vi "SI SetVoltage.vi"(8 "error in (no error)":errorcluster, 10 "Voltage":dbl, 11 "VISA Refnum in":refnum<visa-resource-name>) -> (0 "error out":errorcluster, 3 "String":string)   [LabVIEW 2017]
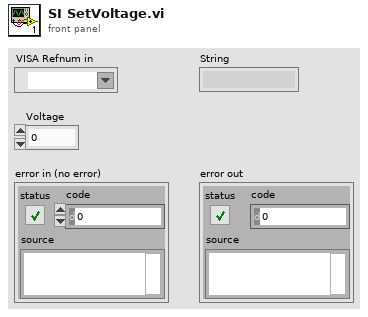
[diagram p1: front panel]
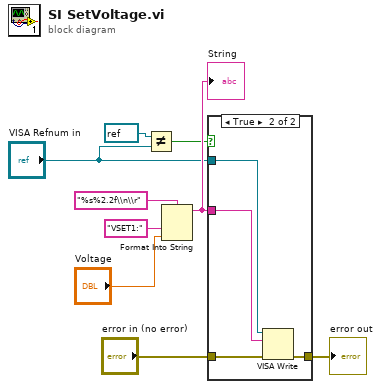
[diagram p0: block diagram]
diagram:
  n1 = Not Equal?(x=refnum<visa-resource-name> refnum ("Laser Port"), y="VISA Refnum in") -> (x != y?=w2:bool)
  n2 = Format Into String(format string="%s%2.2f\\n\\r", "VSET1:", "Voltage") -> (resulting string=w7:string)  [unwired: 2 in, 1 out]
  "String" <- w7
  n3 = case shown="True" w2 {
    tunnel: "VISA Refnum in" -> [_ w14]
    tunnel: "error in (no error)" -> [w10 w13]
    tunnel: [w10 w12] -> w9
    tunnel: w7 -> [_ w11]
    frame False {
    }
    frame True {
      n4 = VISA Write(VISA resource name=w14, write buffer=w11, error in (no error)=w13) -> (error out=w12:errorcluster)  [unwired: 2 out]
    }
  }
  "error out" <- w9
